vi "Zero voltages.vi"(8 "error in":errorcluster, 10 "Channels":string[](array[string]), 11 "Handle in":i32) -> (0 "error out":errorcluster, 3 "Handle out":i32)   [LabVIEW 2018]
panel:
  # "This subVI sets the voltages on the provided TDAC channels to zero"
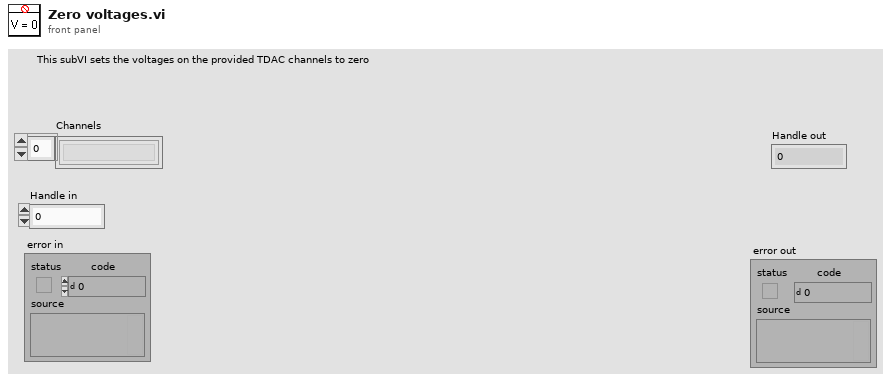
[diagram p1: front panel]
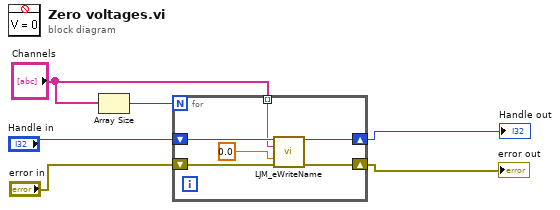
[diagram p0: block diagram]
diagram:
  n1 = Array Size(array="Channels") -> (size(s)=w1:i32)
  n2 = for {
    N: w1 -> [_]
    shift-right: [w10] -> w4
    shift-left: "Handle in" -> [w12]
    shift-right: [w9] -> w3
    shift-left: "error in" -> [w11]
    tunnel: "Channels" -> [w8] mode=indexing
    n3 = call "LJM_eWriteName.vi"("Handle In"=w12, "Name"=w8, "Value"=0.0, "error in"=w11) -> ("Handle Out"=w10:i32, "error out"=w9:errorcluster)  [unwired: 10 in]
  }
  "Handle out" <- w4
  "error out" <- w3
